vi "Day 7.2.vi"(11 "input":string[](array[string])) -> (3 "ouptut part 2":u64)   [LabVIEW 2021]
uses:
  <vilib>/regexp/Match Regular Expression.xnode
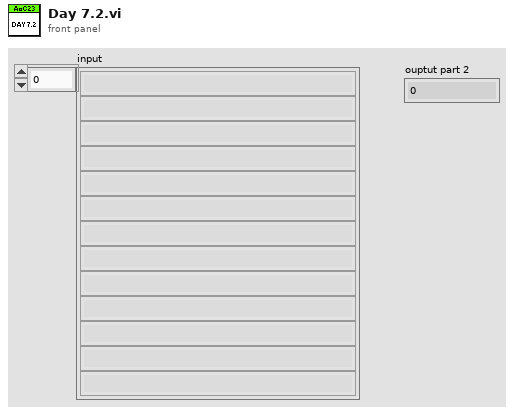
[diagram p1: front panel]
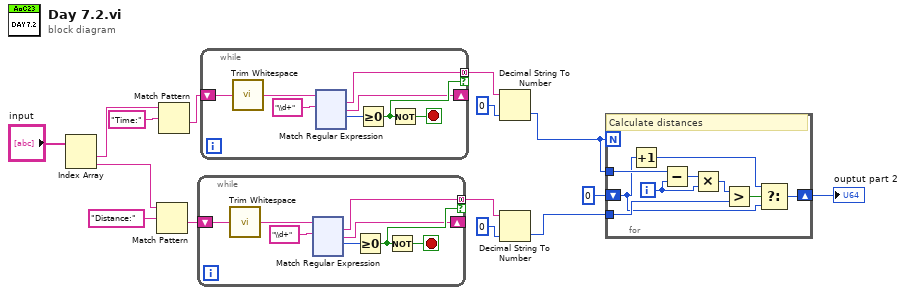
[diagram p0: block diagram]
diagram:
  n1 = Index Array(array="input") -> (element #1=w15:string, element #2=w12:string)  [unwired: 2 in]
  n2 = Match Pattern(string=w12, regular expression="Distance:") -> (after substring=w10:string)  [unwired: 1 in, 3 out]
  n3 = Match Pattern(string=w15, regular expression="Time:") -> (after substring=w11:string)  [unwired: 1 in, 3 out]
  n4 = while {
    tunnel: [w17] -> w7 mode=concatenating if=w20
    shift-right: [w18] -> _
    shift-left: w10 -> [w23]
    stop <- w19 stop-if-true
    n5 = call <vilib>:"Trim Whitespace.vi"("string"=w23) -> ("trimmed string"=w16:string)  [unwired: 1 in]
    n6 = xnode "Match Regular Expression"("input string"=w16, "regular expression"="\\d+") -> ("whole match"=w17:string, "after match"=w18:string, "offset past match"=w21:i32)  [unwired: 4 in, 2 out]
    n7 = Greater Or Equal To 0?(x=w21) -> (x >= 0?=w20:bool)
    n8 = Not(x=w20) -> (.not. x?=w19:bool)
  }
  n9 = while {
    tunnel: [w142] -> w9 mode=concatenating if=w145
    shift-right: [w143] -> _
    shift-left: w11 -> [w148]
    stop <- w144 stop-if-true
    n10 = call <vilib>:"Trim Whitespace.vi"("string"=w148) -> ("trimmed string"=w141:string)  [unwired: 1 in]
    n11 = xnode "Match Regular Expression"("input string"=w141, "regular expression"="\\d+") -> ("whole match"=w142:string, "after match"=w143:string, "offset past match"=w146:i32)  [unwired: 4 in, 2 out]
    n12 = Greater Or Equal To 0?(x=w146) -> (x >= 0?=w145:bool)
    n13 = Not(x=w145) -> (.not. x?=w144:bool)
  }
  n14 = Decimal String To Number(string=w9, default (0L)=u64 0 ("default (0 I32)")) -> (number=w5:u64)  [unwired: 1 in, 1 out]
  n15 = Decimal String To Number(string=w7, default (0L)=u64 0 ("default (0 I32)")) -> (number=w4:u64)  [unwired: 1 in, 1 out]
  n16 = for {
    N: w5 -> [_]
    tunnel: w5 -> [w274]
    tunnel: w4 -> [w270]
    shift-right: [w268] -> w3
    shift-left: u64 0 -> [w266]
    i -> [w272]
    # "Calculate distances"
    n17 = Increment(x=w266) -> (x+1=w267:u64)
    n18 = Subtract(x=w274, y=w272) -> (x-y=w273:u64)
    n19 = Multiply(x=w273, y=w272) -> (x*y=w271:u64)
    n20 = Greater?(x=w271, y=w270) -> (0:w269:bool)
    n21 = Select(t=w267, s=w269, f=w266) -> (s? t:f=w268:u64)
  }
  "ouptut part 2" <- w3
